vi "Update Function UI.vi"(11 "measured_current":dbl) -> (1 "Function":T1, 2 "BG Color":u32, 3 "Font Color":u32)   [LabVIEW 2023]
uses:
  Types/Power Function.ctl
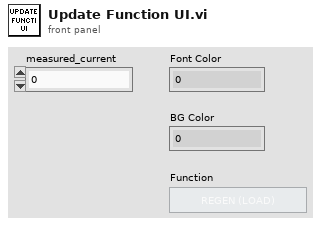
[diagram p1: front panel]
types:
  T1 = typedef "Power Function.ctl" = enum16{"REGEN (LOAD)", "STANDBY", "SUPPLY (SOURCE)"}
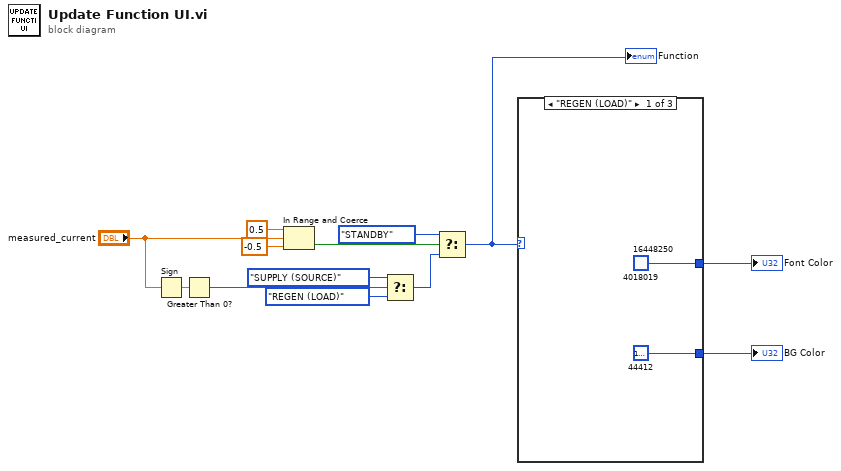
[diagram p0: block diagram]
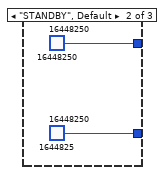
[diagram p2: hidden frame]
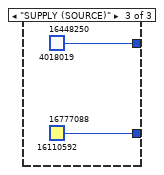
[diagram p3: hidden frame]
diagram:
  n1 = Sign(1:"measured_current") -> (0:w11:dbl)
  n2 = Greater Than 0?(x=w11) -> (x > 0?=w7:bool)
  n3 = In Range and Coerce(upper limit=sgl 0.5, x="measured_current", lower limit=sgl -0.5 ("upper limit")) -> (In Range?=w12:bool)  [unwired: 1 out]
  n4 = Select(t=Power_Function."SUPPLY (SOURCE)" ("FUNCTION"), s=w7, f=Power_Function."REGEN (LOAD)" ("FUNCTION")) -> (s? t:f=w13:T1)
  n5 = Select(t=Power_Function."STANDBY" ("FUNCTION"), s=w12, f=w13) -> (s? t:f=w3:T1)
  "Function" <- w3
  n6 = case shown="\"REGEN (LOAD)\"" w3 {
    tunnel: [u32 4018019 u32 16448250 u32 4018019] -> w2
    tunnel: [u32 44412 u32 1644825 u32 16110592] -> w1
    frame "REGEN (LOAD)" {
      (unwired) u32 16777224
      (unwired) u32 16448250
    }
    frame "STANDBY", Default {
      (unwired) u32 16448250
      (unwired) u32 16448250
    }
    frame "SUPPLY (SOURCE)" {
      (unwired) u32 16448250
      (unwired) u32 16777088
    }
  }
  "Font Color" <- w2
  "BG Color" <- w1
